vi "_CoboltLaser_VI_Tree.vi"   [LabVIEW 2019]
doc: "Use this template to build a VI to use as a subVI."
panel:
  # "Overview of Cobolt Laser drivers in block diagram"
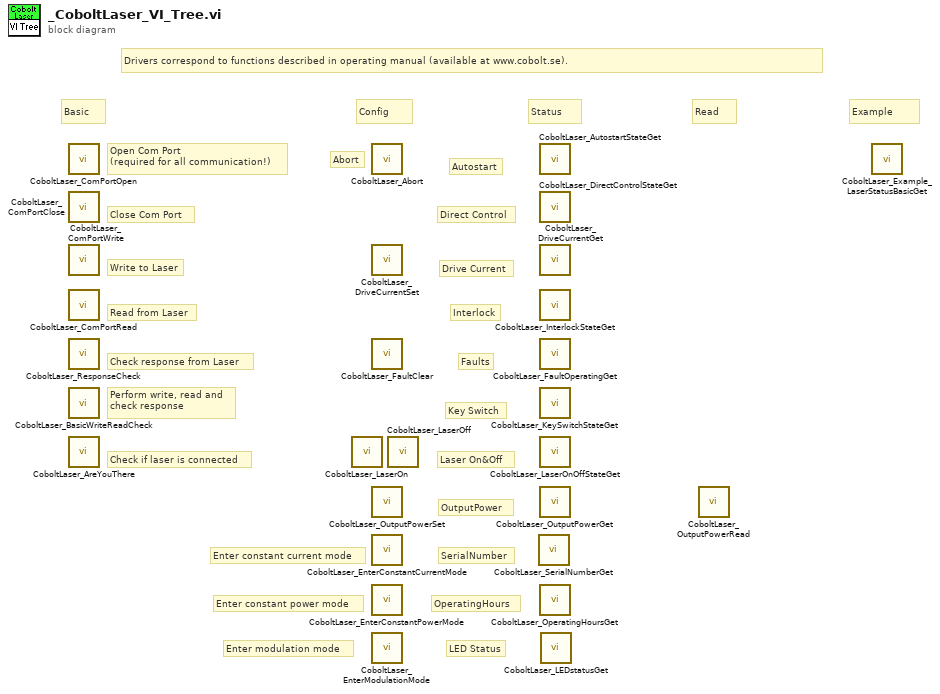
[diagram p0: block diagram]
diagram:
  # "Abort"
  # "Enter modulation mode"
  # "Enter constant power mode"
  # "Enter constant current mode"
  # "Check if laser is connected"
  # "Drivers correspond to functions described in operating manual (available at www.cobolt.se)."
  # "LED Status"
  # "OperatingHours"
  # "SerialNumber"
  # "OutputPower"
  # "Laser On&Off"
  # "Key Switch"
  # "Faults"
  # "Interlock"
  # "Drive Current"
  # "Direct Control"
  # "Autostart"
  # "Perform write, read and\ncheck response"
  # "Check response from Laser"
  # "Read from Laser"
  # "Write to Laser"
  # "Close Com Port"
  # "Open Com Port\n(required for all communication!)"
  # "Example"
  # "Basic"
  # "Read"
  # "Status"
  # "Config"
  n1 = call <userlib>:"CoboltLaser_ComPortOpen.vi"() -> ()  [unwired: 18 in, 2 out]
  n2 = call <userlib>:"CoboltLaser_ComPortClose.vi"() -> ()  [unwired: 19 in, 1 out]
  n3 = call <userlib>:"CoboltLaser_ComPortWrite.vi"() -> ()  [unwired: 18 in, 2 out]
  n4 = call <userlib>:"CoboltLaser_ComPortRead.vi"() -> ()  [unwired: 17 in, 3 out]
  n5 = call <userlib>:"CoboltLaser_ResponseCheck.vi"() -> ()  [unwired: 17 in, 3 out]
  n6 = call <userlib>:"CoboltLaser_BasicWriteReadCheck.vi"() -> ()  [unwired: 24 in, 4 out]
  n7 = call <userlib>:"CoboltLaser_AreYouThere.vi"() -> ()  [unwired: 25 in, 3 out]
  n8 = call <userlib>:"CoboltLaser_LaserOn.vi"() -> ()  [unwired: 24 in, 4 out]
  n9 = call <userlib>:"CoboltLaser_Abort.vi"() -> ()  [unwired: 26 in, 2 out]
  n10 = call <userlib>:"CoboltLaser_DriveCurrentSet.vi"() -> ()  [unwired: 26 in, 2 out]
  n11 = call <userlib>:"CoboltLaser_FaultClear.vi"() -> ()  [unwired: 26 in, 2 out]
  n12 = call <userlib>:"CoboltLaser_OutputPowerSet.vi"() -> ()  [unwired: 26 in, 2 out]
  n13 = call <userlib>:"CoboltLaser_EnterConstantCurrentMode.vi"() -> ()  [unwired: 26 in, 2 out]
  n14 = call <userlib>:"CoboltLaser_EnterConstantPowerMode.vi"() -> ()  [unwired: 26 in, 2 out]
  n15 = call <userlib>:"CoboltLaser_EnterModulationMode.vi"() -> ()  [unwired: 26 in, 2 out]
  n16 = call <userlib>:"CoboltLaser_LaserOff.vi"() -> ()  [unwired: 24 in, 4 out]
  n17 = call <userlib>:"CoboltLaser_SerialNumberGet.vi"() -> ()  [unwired: 24 in, 4 out]
  n18 = call <userlib>:"CoboltLaser_AutostartStateGet.vi"() -> ()  [unwired: 23 in, 5 out]
  n19 = call <userlib>:"CoboltLaser_DirectControlStateGet.vi"() -> ()  [unwired: 25 in, 3 out]
  n20 = call <userlib>:"CoboltLaser_DriveCurrentGet.vi"() -> ()  [unwired: 25 in, 3 out]
  n21 = call <userlib>:"CoboltLaser_InterlockStateGet.vi"() -> ()  [unwired: 25 in, 3 out]
  n22 = call <userlib>:"CoboltLaser_FaultOperatingGet.vi"() -> ()  [unwired: 25 in, 3 out]
  n23 = call <userlib>:"CoboltLaser_KeySwitchStateGet.vi"() -> ()  [unwired: 25 in, 3 out]
  n24 = call <userlib>:"CoboltLaser_LaserOnOffStateGet.vi"() -> ()  [unwired: 23 in, 5 out]
  n25 = call <userlib>:"CoboltLaser_OutputPowerGet.vi"() -> ()  [unwired: 25 in, 3 out]
  n26 = call <userlib>:"CoboltLaser_OperatingHoursGet.vi"() -> ()  [unwired: 25 in, 3 out]
  n27 = call <userlib>:"CoboltLaser_LEDstatusGet.vi"() -> ()  [unwired: 22 in, 6 out]
  n28 = call <userlib>:"CoboltLaser_OutputPowerRead.vi"() -> ()  [unwired: 25 in, 3 out]
  n29 = call <userlib>:"CoboltLaser_Example_LaserStatusBasicGet.vi"() -> ()  [unwired: 27 in, 1 out]
